vi "Read Global Position.vi"(8 "error in (no error)":errorcluster, 11 "GPS in":refnum<class "GPS.lvclass">) -> (0 "error out":errorcluster, 1 "string":string, 2 "GPSReturn":T1 {"UTC Time Stamp" format="%<%.3X>T"; "Longitude" format="%#_12f"; "Latitude" format="%#_12f"}, 3 "GPS out":refnum<class "GPS.lvclass">)   [LabVIEW 2020, in "CTI-Peripheral.lvlib" / "GPS.lvclass"]
uses:
  GPS.lvclass
  DFRobot_Gravity_GNSS/Private/GPSReturn.ctl
  DFRobot_Gravity_GNSS/DFRobot_Gravity_GNSS.lvclass
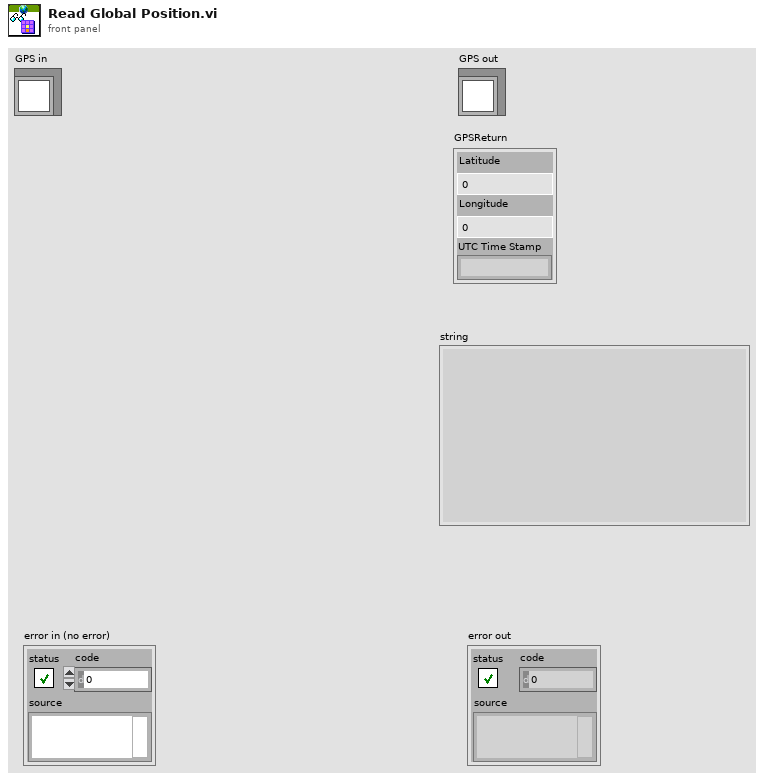
[diagram p1: front panel]
types:
  T1 = typedef "CTI-Peripheral.lvlib/DFRobot_Gravity_GNSS.lvclass/GPSReturn.ctl" = cluster{"Latitude":dbl, "Longitude":dbl, "UTC Time Stamp":timestamp}
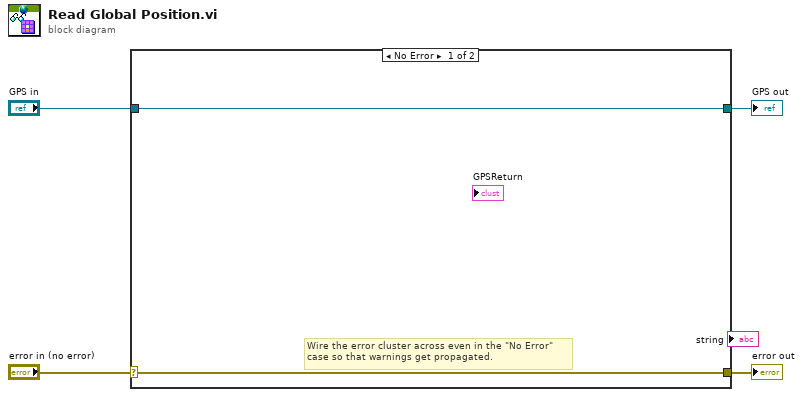
[diagram p0: block diagram]
diagram:
  n1 = case shown="No Error" "error in (no error)" {
    selector: "error in (no error)" -> [w5 w8]
    tunnel: [w5 w8] -> w3
    tunnel: [w6 w7] -> w1
    tunnel: "GPS in" -> [w6 w7]
    frame No Error {
      # "Wire the error cluster across even in the \"No Error\"\ncase so that warnings get propagated."
    }
    frame Error {
    }
  }
  "error out" <- w3
  "GPS out" <- w1
